vi "ICNC Probe.vi"(0 "Axe":u32, 1 "MaxStroke":u32, 2 "FStart":u32, 3 "Decel":u32, 5 "Direction":u32, 7 "InNo":u32, 9 "InValue":i32, 11 "error in (no error)":errorcluster caption="entrée d'erreur (pas d'erreur)", 12 "Speed":u32, 13 "Accel":u32) -> (4 "function return":u32, 15 "error out":errorcluster caption="sortie d'erreur")   [LabVIEW 2012, in "ICNC2.lvlib"]
doc: "DWORD ICNC_Probe(DWORD Axe, DWORD Direction, DWORD InNo, BOOL InValue, DWORD MaxStroke, DWORD Speed, DWORD FStart, DWORD Accel, DWORD Decel);"
uses:
  <userlib>/ICNC/ICNC2.lvlib
  <userlib>/ICNC/ICNC2.dll
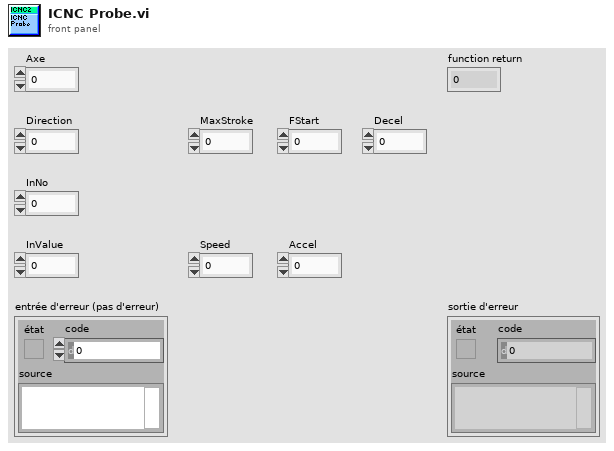
[diagram p1: front panel]
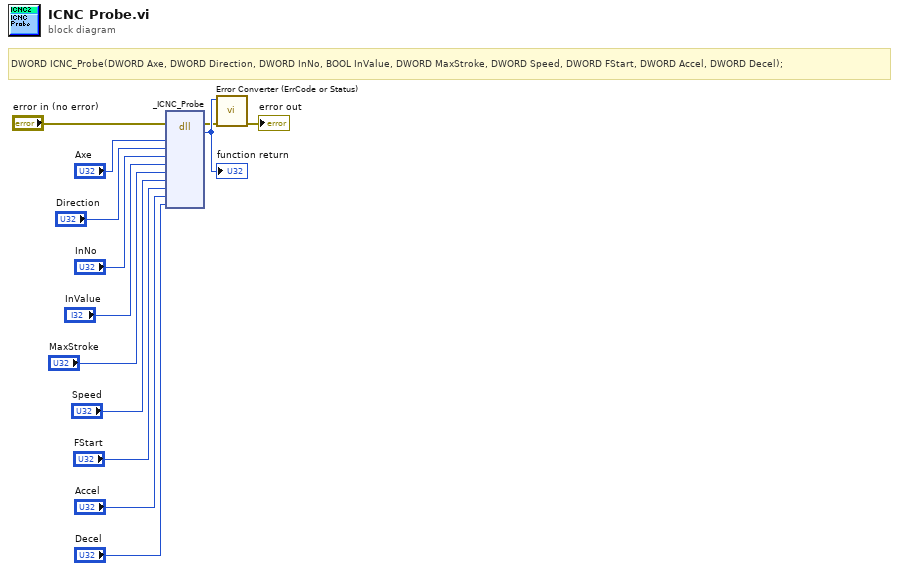
[diagram p0: block diagram]
diagram:
  # "DWORD ICNC_Probe(DWORD Axe, DWORD Direction, DWORD InNo, BOOL InValue, DWORD MaxStroke, DWORD Speed, DWORD FStart, DWORD Accel, DWORD Decel);"
  n1 = dll-call lib="C:/Program Files (x86)/National Instruments/LabVIEW 2012/user.lib/ICNC/ICNC2.*" fn="_ICNC_Probe"(error in="error in (no error)", "Axe"="Axe", "Direction"="Direction", "InNo"="InNo", "InValue"="InValue", "MaxStroke"="MaxStroke", "Speed"="Speed", "FStart"="FStart", "Accel"="Accel", "Decel"="Decel") -> (error out=w2:errorcluster, w13:u32)  [unwired: 11 in, 1 out]
  "function return" <- w13
  n2 = call <userlib>:"Error Converter (ErrCode or Status).vi"("error in (no error)"=w2, "error code"=w13) -> ("error out"=→"error out":errorcluster)  [unwired: 9 in]
